vi "Main.vi"(11 "Module Admin":refnum<class "Delacor_lib_QMH_Cloneable Module Admin.lvclass">) -> ()   [LabVIEW 2021, in "TCP-IP Engine.lvlib"]
doc: "This template is based off of the Queued Message Handler design pattern and the Queued Message Handler project template that ships with LabVIEW.\n\nThe main difference is that the queue is private to this module and communication between modules is performed via Broadcast and Request events.\n\nRequest events are wrapped in public API methods and are handled in the Event Handling Loop (EHL) of this VI. Any module can register for Broadcast events sent by this module. The EHL generates messages based on user interface actions.\n\nThe Message Handling Loop (MHL) processes messages generated by the EHL, or by other messages. The messages are string values, so new messages can be added easily to the Message Cases case structure in the MHL. Each message cluster can also provide an optional value for Message Data, which is a variant that can be converted to whatever message-specific data is required.\n_____\nBased on DQMH Project Template 7.0.1.1316."
uses:
  TCP-IP Engine.lvlib
  <vilib>/Delacor/Delacor QMH/Libraries/Cloneable Module Admin_class/Delacor_lib_QMH_Cloneable Module Admin.lvclass
  C:/Program Files (x86)/National Instruments/LabVIEW 2024/vi.lib/Delacor/Delacor QMH/Libraries/Module Admin_class/Delacor_lib_QMH_Module Admin.lvclass
  Module Data--cluster.ctl
  TCP-Open Connection Argument--cluster.ctl
  <vilib>/Delacor/Delacor QMH/Libraries/Message Queue_class/Delacor_lib_QMH_Message Queue.lvclass/Delacor_lib_QMH_Message Queue.ctl
  <vilib>/Delacor/Delacor QMH/Libraries/Cloneable Module Admin_class/Delacor_lib_QMH_Cloneable Module Admin.lvclass/Delacor_lib_QMH_Cloneable Module Admin.ctl
  Stop Argument--cluster.ctl
  <vilib>/Delacor/Delacor QMH/Libraries/Module Admin_class/Delacor_lib_QMH_Module Admin.lvclass/Delacor_lib_QMH_Module Admin.ctl
  Read TCP Data Argument--cluster.ctl
  TCP-Write Argument--cluster.ctl
  TCP-Close Connection Argument--cluster.ctl
  <vilib>/Utility/miscctls.llb/LVPointTypeDef.ctl
  <vilib>/Delacor/Delacor QMH/Libraries/Message Queue_class/Delacor_lib_QMH_Enqueue Message (Single).vi
  <vilib>/Delacor/Delacor QMH/Libraries/Cloneable Module Admin_class/Delacor_lib_QMH_Get Module ID.vi
  <vilib>/Delacor/Delacor QMH/Libraries/Module Admin_class/Delacor_lib_QMH_Get External Launch.vi
  <vilib>/Delacor/Delacor QMH/Libraries/Message Queue_class/Delacor_lib_QMH_Message Queue.lvclass
panel:
  out "x >= y?":bool
  out "error out":errorcluster
  out "Status":string
  in  "Simulate EHL Error":bool
  in  "Simulate MHL Error":bool
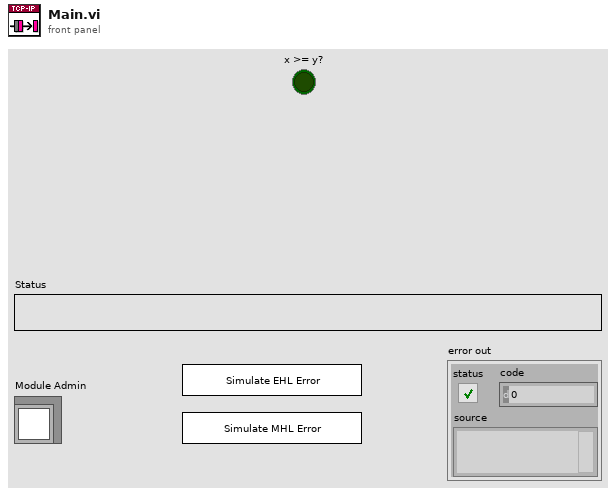
[diagram p1: front panel]
types:
  T1 = typedef "TCP-IP Engine.lvlib/Request Events--cluster.ctl" = cluster{"Stop Module":refnum<user-event>, "Show Panel":refnum<user-event>, "Hide Panel":refnum<user-event>, "Show Diagram":refnum<user-event>, "Get Module Execution Status":refnum<user-event>, "TCP-Open Connection":refnum<user-event>, "Read TCP Data":refnum<user-event>, "TCP-Write":refnum<user-event>, "TCP-Close Connection":refnum<user-event>}
  T2 = typedef "TCP-IP Engine.lvlib/Module Data--cluster.ctl" = cluster{"Status":string, "TCP-ID":refnum<k5>, "TCP-Open Connection Argument":T3, "OC Err Time":timestamp}
  T3 = typedef "TCP-IP Engine.lvlib/TCP-Open Connection Argument--cluster.ctl" = cluster{"Module ID":i32, "local port (0)":u16, "timeout ms (60000)":i32, "remote port ":u16, "address":string}
  T4 = enum32{"invalid lock state", "Not Locked", "Locked (No Password)", "Password-protected"}
  T5 = typedef "TCP-IP Engine.lvlib/Stop Argument--cluster.ctl" = cluster{"Module ID":i32, "Origin":string, "Exit via Stop Module Req?":bool, "Wait for Module to stop?":bool}
  T6 = typedef "TCP-IP Engine.lvlib/Read TCP Data Argument--cluster.ctl" = cluster{"Module ID":i32, "mode (standard)":enum16{"Standard", "Buffered", "CRLF", "Immediate"}, "timeout ms (25000)":i32, "bytes to read":i32}
  T7 = typedef "TCP-IP Engine.lvlib/TCP-Write Argument--cluster.ctl" = cluster{"Module ID":i32, "timeout ms (25000)":i32, "data in":string}
  T8 = typedef "TCP-IP Engine.lvlib/TCP-Close Connection Argument--cluster.ctl" = cluster{"Module ID":i32, "abort (F)":bool}
  T9 = typedef "LVPointTypeDef.ctl" = cluster{"Horizontal":i16, "Vertical":i16}
  T10 = enum32{"Invalid", "Standard", "Closed", "Hidden", "Minimized", "Maximized"}
  T11 = enum16{"big-endian, network order", "native, host order", "little-endian"}
  T12 = enum16{"Standard", "Buffered", "CRLF", "Immediate"}
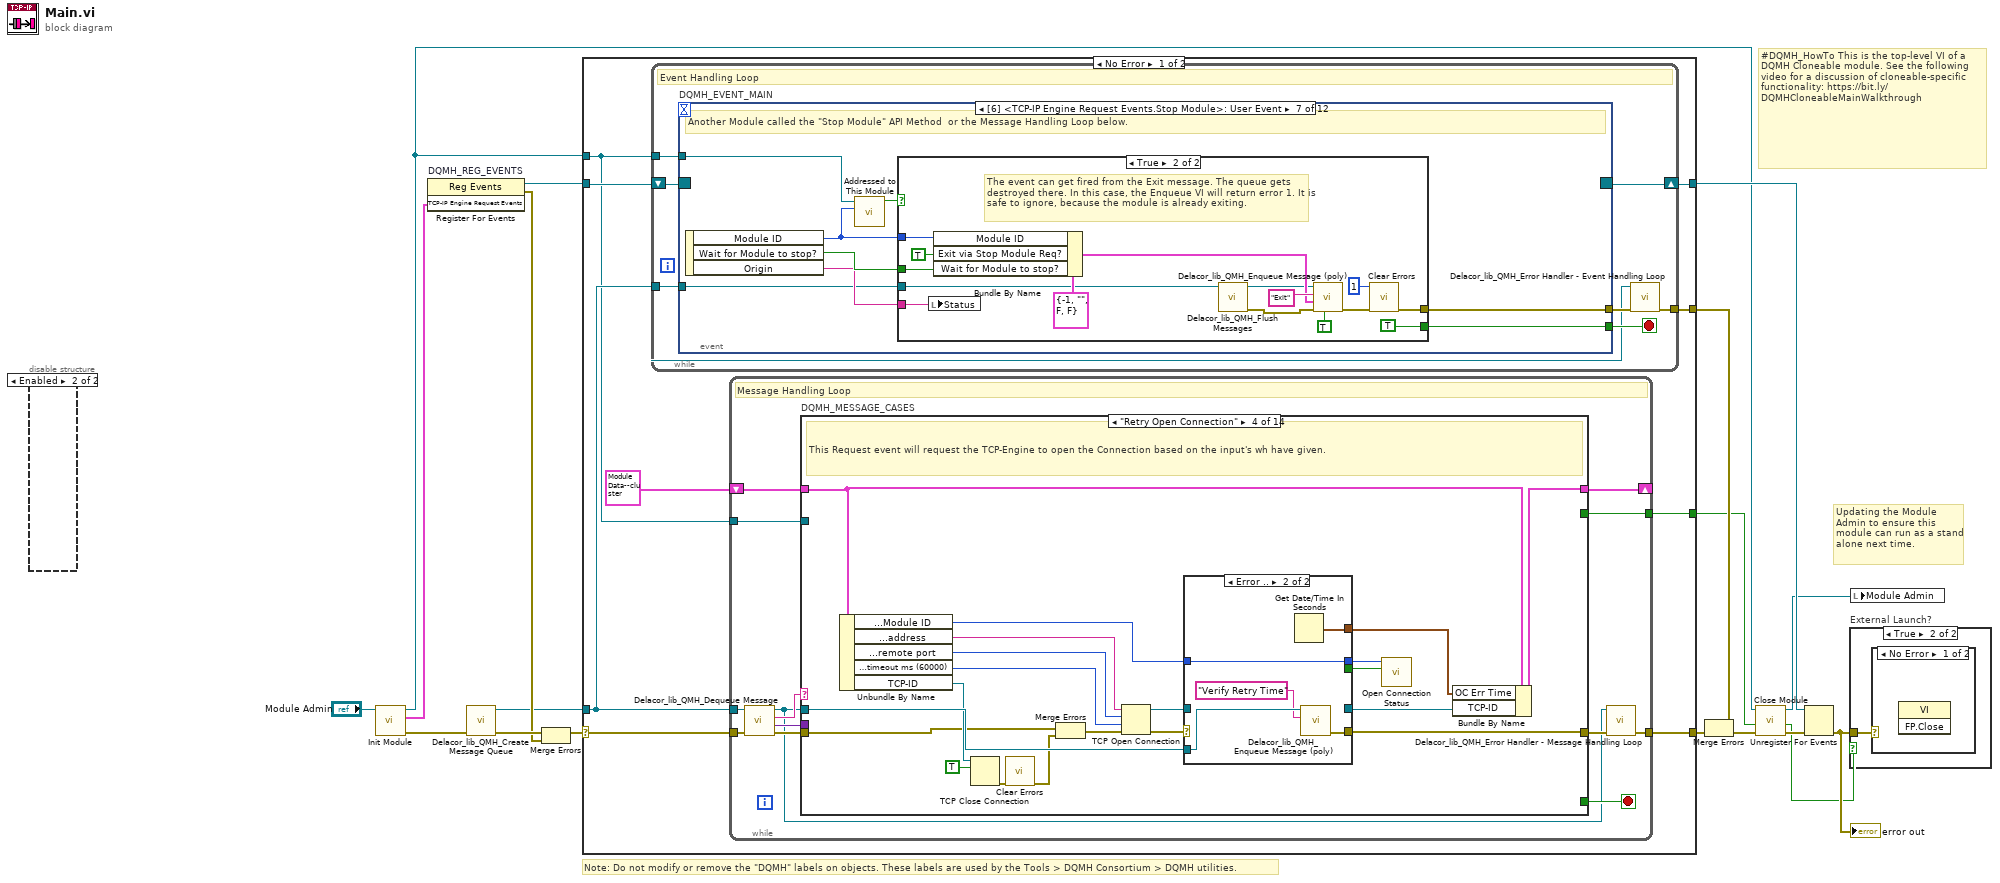
[diagram p0: block diagram]
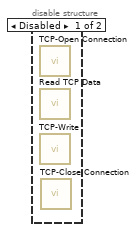
[diagram p2: hidden frame]
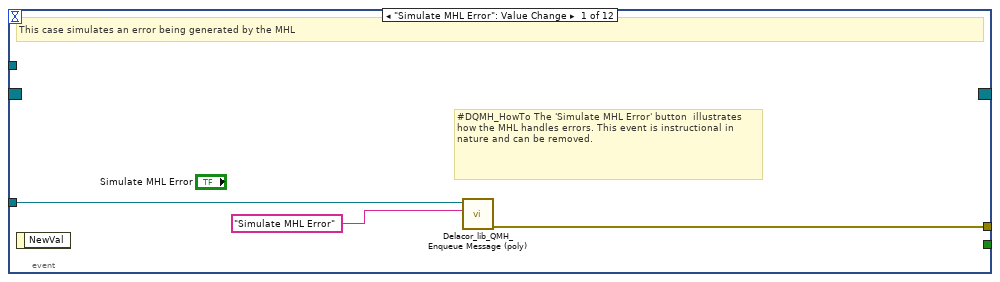
[diagram p3: hidden frame]
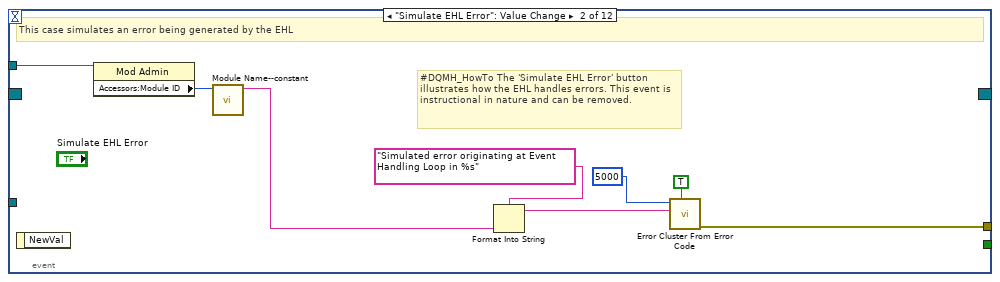
[diagram p4: hidden frame]
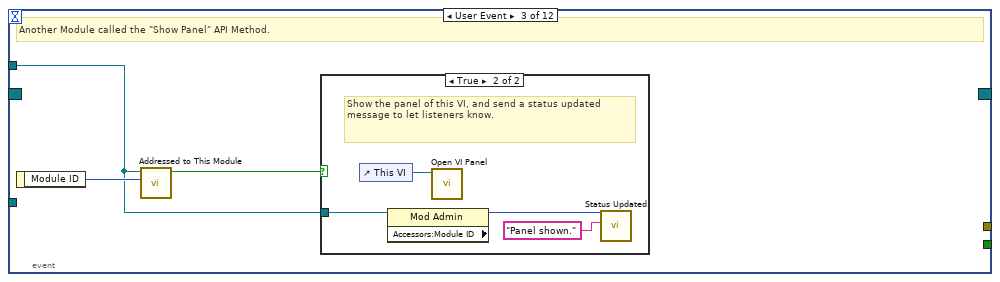
[diagram p5: hidden frame]
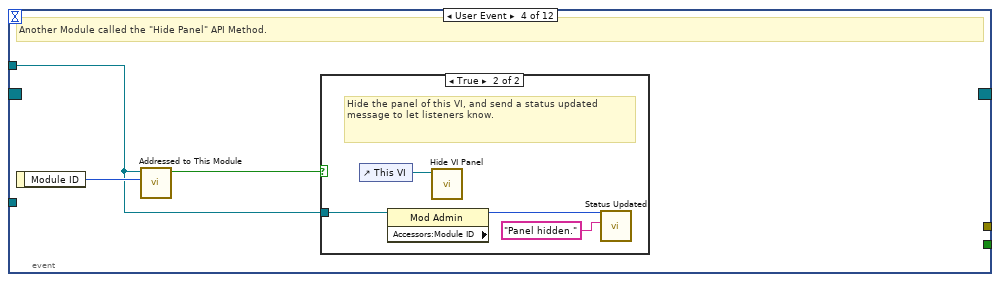
[diagram p7: hidden frame]
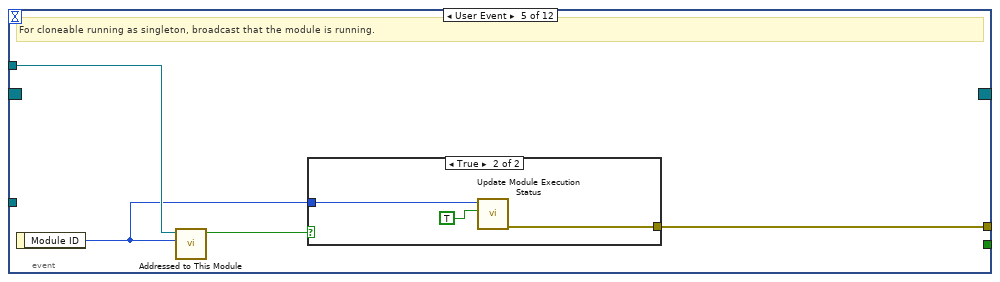
[diagram p9: hidden frame]
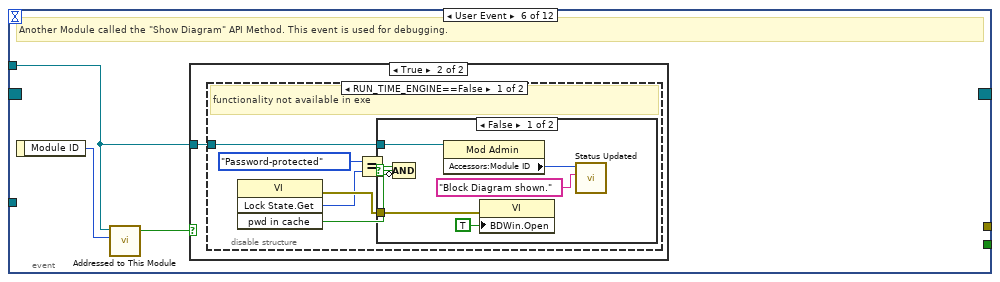
[diagram p11: hidden frame]
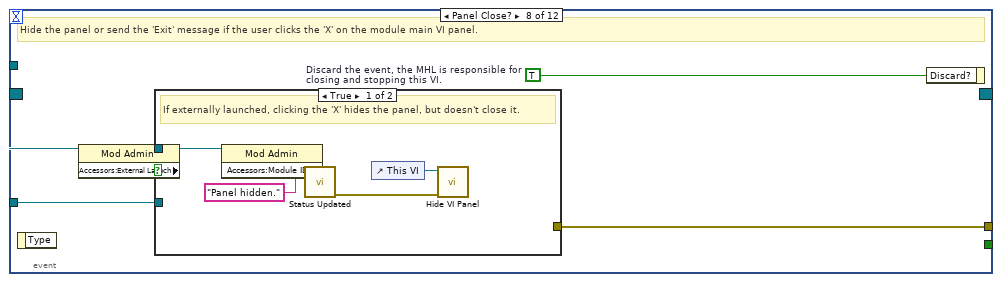
[diagram p16: hidden frame]
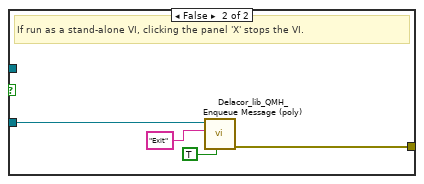
[diagram p17: hidden frame]
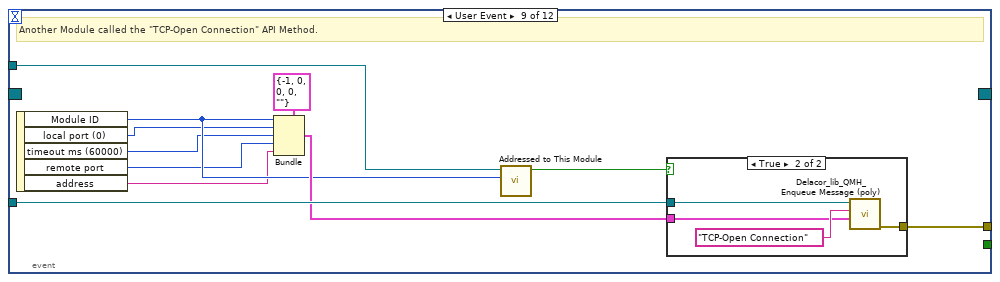
[diagram p18: hidden frame]
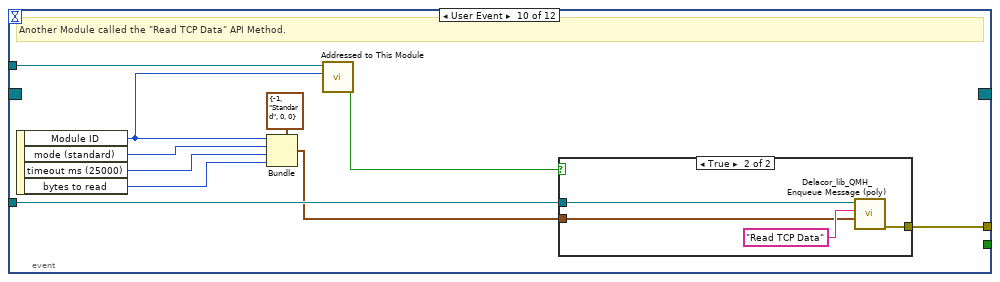
[diagram p20: hidden frame]
diagram:
  # "#DQMH_HowTo This is the top-level VI of a DQMH Cloneable module. See the following video for a discussion of cloneable-specific functionality: https://bit.ly/DQMHCloneableMainWalkthrough"
  # "Note: Do not modify or remove the \"DQMH\" labels on objects. These labels are used by the Tools > DQMH Consortium > DQMH utilities."
  # "Updating the Module Admin to ensure this module can run as a stand alone next time."
  n1 = disable-structure shown="Enabled" {
    frame Disabled {
      n2 = call "TCP-Open Connection.vi"() -> ()  [unwired: 11 in, 1 out]
      n3 = call "Read TCP Data.vi"() -> ()  [unwired: 11 in, 1 out]
      n4 = call "TCP-Write.vi"() -> ()  [unwired: 11 in, 1 out]
      n5 = call "TCP-Close Connection.vi"() -> ()  [unwired: 11 in, 1 out]
    }
    frame Enabled {
    }
  }
  n6 = call "Init Module.vi"("Cloneable Module Admin in"="Module Admin") -> ("error out"=w15:errorcluster, "TCP-IP Engine Request Events"=w7:T1, "Cloneable Module Admin out"=w4:refnum<class "Delacor_lib_QMH_Cloneable Module Admin.lvclass">)  [unwired: 8 in]
  n7 = register-events "DQMH_REG_EVENTS"(w7) -> (reference out=w8:refnum<event-registration>, error out=w10:errorcluster)  [unwired: 2 in]
  n8 = call <vilib>:"Delacor_lib_QMH_Create Message Queue.vi"("error in"=w15) -> ("error out"=w12:errorcluster, "Message Queue"=w6:refnum<class "Delacor_lib_QMH_Message Queue.lvclass">)  [unwired: 9 in]
  n9 = Merge Errors(w12, w10) -> (w11:errorcluster)
  n10 = case shown="No Error" w11 {
    selector: w11 -> [w25 w458]
    tunnel: [w27 w457] -> w16
    tunnel: [w24 w456] -> w9
    tunnel: w8 -> [w22 w456]
    tunnel: w6 -> [w21 w449]
    tunnel: [w26 _] -> w17
    tunnel: w4 -> [w20 w452]
    tunnel: [w19 _] -> w2
    frame No Error {
      n11 = while {
        tunnel: w21 -> [w28]
        shift-right: [w31] -> w24
        shift-left: w22 -> [w32]
        tunnel: [w33] -> w26
        tunnel: w20 -> [w29]
        stop <- w30 stop-if-true
        # "Event Handling Loop"
        n12 = event "DQMH_EVENT_MAIN" shown="[6] <TCP-IP Engine Request Events.Stop Module>: User Event" {
          selector: w32 -> [_ _ _ _ _ _ _ _ _ _ _ _]
          dyn-events: [_ _ _ _ _ _ _ _ _ _ _ _] -> w31
          timeout: _ -> [_ _ _ _ _ _ _ _ _ _ _ _]
          tunnel: [_ _ _ _ _ _ w87 _ _ _ _ _] -> w30
          tunnel: w28 -> [w36 _ _ _ _ _ w83 w108 w131 w145 w158 w171]
          tunnel: [w37 w45 _ _ w63 _ w90 w111 w121 w136 w150 w164] -> w34
          tunnel: w29 -> [_ w44 w46 w53 w61 w67 w89 w109 w129 w143 w156 w169]
          event "Simulate MHL Error": Value Change {
            # "#DQMH_HowTo The 'Simulate MHL Error' button  illustrates how the MHL handles errors. This event is instructional in nature and can be removed."
            # "This case simulates an error being generated by the MHL"
            n13 = event-data() -> ()  [unwired: 1 in, 1 out]
            n14 = call-poly <vilib>:"Delacor_lib_QMH_Enqueue Message (poly).vi"("Message"="Simulate MHL Error", "Message Queue in"=w36) -> ("error out"=w37:errorcluster)  [unwired: 8 in, 1 out]
          }
          event "Simulate EHL Error": Value Change {
            # "#DQMH_HowTo The 'Simulate EHL Error' button  illustrates how the EHL handles errors. This event is instructional in nature and can be removed."
            # "This case simulates an error being generated by the EHL"
            n15 = event-data() -> ()  [unwired: 1 in, 1 out]
            n16 = property on="Property Node" class="Mod Admin"(reference=w44) -> ("Accessors:Module ID"=w43:i32)  [unwired: 1 in, 2 out]
            n17 = call "Module Name--constant.vi"("Module ID"=w43) -> ("Module Name"=w38:string)  [unwired: 10 in]
            n18 = Format Into String(format string="Simulated error originating at Event Handling Loop in %s", w38) -> (resulting string=w41:string)  [unwired: 2 in, 1 out]
            n19 = call <vilib>:"Error Cluster From Error Code.vi"("show call chain? (False)"=TRUE, "error message (\"\")"=w41, "error code (0)"=5000) -> ("error out"=w45:errorcluster)  [unwired: 6 in]
          }
          event User Event {
            # "Another Module called the \"Show Panel\" API Method."
            n20 = event-data() -> ("Module ID"=w47:i32)  [unwired: 1 in]
            n21 = call "Addressed to This Module.vi"("Module ID from Argument"=w47, "Module Admin"=w46) -> ("Addressed to this instance?"=w48:bool)  [unwired: 8 in, 1 out]
            n22 = case shown="True" w48 {
              tunnel: w46 -> [_ w50]
              frame False {
              }
              frame True {
                # "Show the panel of this VI, and send a status updated message to let listeners know."
                n23 = control-ref of="This VI"() -> (w52:refnum<vi>)
                n24 = property on="Property Node" class="Mod Admin"(reference=w50) -> ("Accessors:Module ID"=w49:i32)  [unwired: 1 in, 2 out]
                n25 = call "Open VI Panel.vi"("VI"=w52) -> ()  [unwired: 10 in, 1 out]
                n26 = call "Status Updated.vi"("Status"="Panel shown." ("format string"), "Module ID"=w49) -> ()  [unwired: 9 in, 1 out]
              }
            }
          }
          event User Event {
            # "Another Module called the \"Hide Panel\" API Method."
            n27 = event-data() -> ("Module ID"=w54:i32)  [unwired: 1 in]
            n28 = call "Addressed to This Module.vi"("Module ID from Argument"=w54, "Module Admin"=w53) -> ("Addressed to this instance?"=w55:bool)  [unwired: 8 in, 1 out]
            n29 = case shown="True" w55 {
              tunnel: w53 -> [_ w57]
              frame False {
              }
              frame True {
                # "Hide the panel of this VI, and send a status updated message to let listeners know."
                n30 = control-ref of="This VI"() -> (w59:refnum<vi>)
                n31 = property on="Property Node" class="Mod Admin"(reference=w57) -> ("Accessors:Module ID"=w56:i32)  [unwired: 1 in, 2 out]
                n32 = call "Hide VI Panel.vi"("VI"=w59) -> ()  [unwired: 10 in, 1 out]
                n33 = call "Status Updated.vi"("Status"="Panel hidden." ("format string"), "Module ID"=w56) -> ()  [unwired: 9 in, 1 out]
              }
            }
          }
          event User Event {
            # "For cloneable running as singleton, broadcast that the module is running."
            n34 = event-data() -> ("Module ID"=w60:i32)  [unwired: 1 in]
            n35 = call "Addressed to This Module.vi"("Module ID from Argument"=w60, "Module Admin"=w61) -> ("Addressed to this instance?"=w62:bool)  [unwired: 8 in, 1 out]
            n36 = case shown="True" w62 {
              tunnel: [_ w66] -> w63
              tunnel: w60 -> [_ w65]
              frame False {
              }
              frame True {
                n37 = call "Update Module Execution Status.vi"("Running?"=TRUE, "Module ID"=w65) -> ("error out"=w66:errorcluster)  [unwired: 9 in]
              }
            }
          }
          event User Event {
            # "Another Module called the \"Show Diagram\" API Method. This event is used for debugging."
            n38 = event-data() -> ("Module ID"=w68:i32)  [unwired: 1 in]
            n39 = call "Addressed to This Module.vi"("Module ID from Argument"=w68, "Module Admin"=w67) -> ("Addressed to this instance?"=w69:bool)  [unwired: 8 in, 1 out]
            n40 = case shown="True" w69 {
              tunnel: w67 -> [_ w70]
              frame False {
              }
              frame True {
                n41 = disable-structure shown="RUN_TIME_ENGINE==False" {
                  disable-tunnel: w70 -> [w71 _]
                  frame condition #0 (active) {
                    # "functionality not available in exe"
                    n42 = invoke on="Invoke Node" class="VI" method="Lock State.Get"() -> (error out=w77:errorcluster, "Get Lock State"=w76:T4, "pwd in cache"=w73:bool)  [unwired: 4 in, 1 out]
                    n43 = Equal?(x=T4."Password-protected", y=w76) -> (x = y?=w74:bool)
                    n44 = Compound Arithmetic op=AND(w74, invert w73) -> (w72:bool)
                    n45 = case shown="False" w72 {
                      tunnel: w77 -> [w82 _]
                      tunnel: w71 -> [w79 _]
                      frame False {
                        n46 = property on="Property Node" class="Mod Admin"(reference=w79) -> ("Accessors:Module ID"=w78:i32)  [unwired: 1 in, 2 out]
                        n47 = property on="Property Node" class="VI"(error in=w82, "BDWin.Open"=TRUE ("Block Diagram Window:Open")) -> ()  [unwired: 1 in, 2 out]
                        n48 = call "Status Updated.vi"("Status"="Block Diagram shown." ("format string"), "Module ID"=w78) -> ()  [unwired: 9 in, 1 out]
                      }
                      frame True {
                        # "Password-protected VI, and the password is not in the cache. Do not show the diagram."
                      }
                    }
                  }
                  frame condition #1 {
                  }
                }
              }
            }
          }
          event User Event {
            # "Another Module called the \"Stop Module\" API Method  or the Message Handling Loop below."
            n49 = event-data() -> ("Module ID"=w85:i32, "Wait for Module to stop?"=w86:bool, "Origin"=w84:string)  [unwired: 1 in]
            n50 = call "Addressed to This Module.vi"("Module ID from Argument"=w85, "Module Admin"=w89) -> ("Addressed to this instance?"=w88:bool)  [unwired: 8 in, 1 out]
            n51 = case shown="True" w88 {
              tunnel: [_ w104] -> w90
              tunnel: w83 -> [_ w93]
              tunnel: [_ TRUE] -> w87
              tunnel: w86 -> [_ w96]
              tunnel: w85 -> [_ w98]
              tunnel: w84 -> [_ w94]
              frame False {
              }
              frame True {
                # "The event can get fired from the Exit message. The queue gets destroyed there. In this case, the Enqueue VI will return error 1. It is safe to ignore, because the module is already exiting."
                n52 = local write "Status"(w94) -> ()
                n53 = Bundle By Name(cluster=T5 {"Module ID"=-1, "Origin"="", "Exit via Stop Module Req?"=FALSE, "Wait for Module to stop?"=FALSE} ("Stop Argument"), "Module ID"=w98, "Exit via Stop Module Req?"=TRUE, "Wait for Module to stop?"=w96) -> (w95:T5)
                n54 = call-dynamic "Delacor_lib_QMH_Flush Messages.vi"("Message Queue in"=w93) -> ("error out"=w91:errorcluster, "Message Queue out"=w92:refnum<class "Delacor_lib_QMH_Message Queue.lvclass">)  [unwired: 7 in, 2 out]
                n55 = call-poly <vilib>:"Delacor_lib_QMH_Enqueue Message (poly).vi"("Priority Message? (F)"=TRUE, "error in"=w91, "Message Data"=w95, "Message"="Exit", "Message Queue in"=w92) -> ("error out"=w105:errorcluster)  [unwired: 5 in, 1 out]
                n56 = call <vilib>:"Clear Errors.vi"("error in (no error)"=w105, "specific error code to clear (0: all)"=1) -> ("error out"=w104:errorcluster)  [unwired: 4 in, 1 out]
              }
            }
          }
          event Panel Close? {
            w110 = TRUE  # Discard the event, the MHL is responsible for closing and stopping this VI.
            # "Hide the panel or send the 'Exit' message if the user clicks the 'X' on the module main VI panel."
            n57 = event-data() -> ()  [unwired: 1 in, 1 out]
            n58 = property on="Property Node" class="Mod Admin"(reference=w109) -> (reference out=w106:refnum<class "Delacor_lib_QMH_Cloneable Module Admin.lvclass">, "Accessors:External Launch"=w107:bool)  [unwired: 1 in, 1 out]
            n59 = case shown="True" w107 {
              tunnel: w108 -> [_ w119]
              tunnel: [_ w120] -> w111
              tunnel: w106 -> [w114 _]
              frame True {
                # "If externally launched, clicking the 'X' hides the panel, but doesn't close it."
                n60 = property on="Property Node" class="Mod Admin"(reference=w114) -> ("Accessors:Module ID"=w113:i32)  [unwired: 1 in, 2 out]
                n61 = call "Status Updated.vi"("Status"="Panel hidden." ("format string"), "Module ID"=w113) -> ("error out"=w112:errorcluster)  [unwired: 9 in]
                n62 = control-ref of="This VI"() -> (w116:refnum<vi>)
                n63 = call "Hide VI Panel.vi"("error in"=w112, "VI"=w116) -> ()  [unwired: 9 in, 1 out]
              }
              frame False {
                # "If run as a stand-alone VI, clicking the panel 'X' stops the VI."
                n64 = call-poly <vilib>:"Delacor_lib_QMH_Enqueue Message (poly).vi"("Priority Message? (F)"=TRUE, "Message"="Exit", "Message Queue in"=w119) -> ("error out"=w120:errorcluster)  [unwired: 7 in, 1 out]
              }
            }
            n65 = event-data ("Event Filter Node")("Discard?"=w110) -> ()  [unwired: 1 in, 1 out]
          }
          event User Event {
            # "Another Module called the \"TCP-Open Connection\" API Method."
            n66 = event-data() -> ("Module ID"=w126:i32, "local port (0)"=w125:u16, "timeout ms (60000)"=w124:i32, "remote port"=w123:u16, "address"=w122:string)  [unwired: 1 in]
            n67 = Bundle(cluster=T3 {"Module ID"=-1, "local port (0)"=0, "timeout ms (60000)"=0, "remote port "=0, "address"=""} ("TCP-Open Connection Argument"), "Module ID"=w126, "local port (0)"=w125, "timeout ms (60000)"=w124, "remote port"=w123, "address"=w122) -> (w127:T3)
            n68 = call "Addressed to This Module.vi"("Module ID from Argument"=w126, "Module Admin"=w129) -> ("Addressed to this instance?"=w130:bool)  [unwired: 8 in, 1 out]
            n69 = case shown="True" w130 {
              tunnel: w131 -> [_ w135]
              tunnel: w127 -> [_ w133]
              tunnel: [_ w132] -> w121
              frame False {
              }
              frame True {
                n70 = call-poly <vilib>:"Delacor_lib_QMH_Enqueue Message (poly).vi"("Message Data"=w133, "Message"="TCP-Open Connection", "Message Queue in"=w135) -> ("error out"=w132:errorcluster)  [unwired: 7 in, 1 out]
              }
            }
          }
          event User Event {
            # "Another Module called the \"Read TCP Data\" API Method."
            n71 = event-data() -> ("Module ID"=w140:i32, "mode (standard)"=w139:T12, "timeout ms (25000)"=w138:i32, "bytes to read"=w137:i32)  [unwired: 1 in]
            n72 = Bundle(cluster=T6 {"Module ID"=-1, "mode (standard)"=enum."Standard", "timeout ms (25000)"=0, "bytes to read"=0} ("Read TCP Data Argument"), "Module ID"=w140, "mode (standard)"=w139, "timeout ms (25000)"=w138, "bytes to read"=w137) -> (w141:T6)
            n73 = call "Addressed to This Module.vi"("Module ID from Argument"=w140, "Module Admin"=w143) -> ("Addressed to this instance?"=w144:bool)  [unwired: 8 in, 1 out]
            n74 = case shown="True" w144 {
              tunnel: w145 -> [_ w149]
              tunnel: w141 -> [_ w147]
              tunnel: [_ w146] -> w136
              frame False {
              }
              frame True {
                n75 = call-poly <vilib>:"Delacor_lib_QMH_Enqueue Message (poly).vi"("Message Data"=w147, "Message"="Read TCP Data", "Message Queue in"=w149) -> ("error out"=w146:errorcluster)  [unwired: 7 in, 1 out]
              }
            }
          }
          event User Event {
            # "Another Module called the \"TCP-Write\" API Method."
            n76 = event-data() -> ("Module ID"=w153:i32, "timeout ms (25000)"=w152:i32, "data in"=w151:string)  [unwired: 1 in]
            n77 = Bundle(cluster=T7 {"Module ID"=-1, "timeout ms (25000)"=0, "data in"=""} ("TCP-Write Argument"), "Module ID"=w153, "timeout ms (25000)"=w152, "data in"=w151) -> (w154:T7)
            n78 = call "Addressed to This Module.vi"("Module ID from Argument"=w153, "Module Admin"=w156) -> ("Addressed to this instance?"=w157:bool)  [unwired: 8 in, 1 out]
            n79 = case shown="True" w157 {
              tunnel: w158 -> [_ w163]
              tunnel: w154 -> [_ w161]
              tunnel: [_ w160] -> w150
              frame False {
              }
              frame True {
                n80 = call-poly <vilib>:"Delacor_lib_QMH_Enqueue Message (poly).vi"("Priority Message? (F)"=TRUE, "Message Data"=w161, "Message"="TCP-Write", "Message Queue in"=w163) -> ("error out"=w160:errorcluster)  [unwired: 6 in, 1 out]
              }
            }
          }
          event User Event {
            # "Another Module called the \"TCP-Close Connection\" API Method."
            n81 = event-data() -> ("Module ID"=w166:i32, "abort (F)"=w165:bool)  [unwired: 1 in]
            n82 = Bundle(cluster=T8 {"Module ID"=-1, "abort (F)"=FALSE} ("TCP-Close Connection Argument"), "Module ID"=w166, "abort (F)"=w165) -> (w167:T8)
            n83 = call "Addressed to This Module.vi"("Module ID from Argument"=w166, "Module Admin"=w169) -> ("Addressed to this instance?"=w170:bool)  [unwired: 8 in, 1 out]
            n84 = case shown="True" w170 {
              tunnel: w171 -> [_ w175]
              tunnel: w167 -> [_ w173]
              tunnel: [_ w172] -> w164
              frame False {
              }
              frame True {
                n85 = call-poly <vilib>:"Delacor_lib_QMH_Enqueue Message (poly).vi"("Message Data"=w173, "Message"="TCP-Close Connection", "Message Queue in"=w175) -> ("error out"=w172:errorcluster)  [unwired: 7 in, 1 out]
              }
            }
          }
        }
        n86 = call-dynamic "Delacor_lib_QMH_Error Handler - Event Handling Loop.vi"("error in"=w34, "Message Queue in"=w28) -> ("dup error in"=w33:errorcluster)  [unwired: 8 in, 1 out]
      }
      n87 = while {
        tunnel: w21 -> [w176]
        shift-right: [w183] -> _
        shift-left: T2 {"Status"="", "TCP-ID"=refnum, "TCP-Open Connection Argument"={"Module ID"=-1, "local port (0)"=0, "timeout ms (60000)"=0, "remote port "=0, "address"=""}, "OC Err Time"=timestamp(0 s since 1904-01-01)} ("Data Cluster") -> [w184]
        tunnel: w25 -> [w187]
        tunnel: [w185] -> w27
        tunnel: w20 -> [w178]
        tunnel: [w177] -> w19
        stop <- w182 stop-if-true
        # "Message Handling Loop"
        n88 = call-dynamic "Delacor_lib_QMH_Dequeue Message.vi"("error in"=w187, "Message Queue in"=w176) -> ("error out"=w186:errorcluster, "Message Data"=w180:variant, "Message"=w181:string, "Message Queue out"=w179:refnum<class "Delacor_lib_QMH_Message Queue.lvclass">)  [unwired: 6 in]
        n89 = case "DQMH_MESSAGE_CASES" shown="\"Retry Open Connection\"" w181 {
          selector: w181 -> [_ _ _ _ _ _ _ _ _ _ _ _ _ w438]
          tunnel: w179 -> [_ _ w213 w247 w276 _ _ _ w369 _ w390 _ w430 _]
          tunnel: w186 -> [w207 w211 w230 w242 w288 w349 w363 w366 w370 w387 w399 w416 w436 w447]
          tunnel: [w205 w211 w220 w254 w283 w343 w358 w365 w378 w387 w395 w415 w431 w448] -> w188
          tunnel: w184 -> [w198 w210 w223 w248 w279 w345 w356 w364 w377 w386 w394 w413 w420 w445]
          tunnel: [w197 w210 w222 w256 w278 w344 w356 w364 w377 w386 w394 w413 w420 w445] -> w183
          tunnel: [_ _ _ _ _ _ _ _ _ _ _ _ w429 _] -> w182
          tunnel: w180 -> [_ _ w229 _ w287 w348 w362 _ _ _ w393 _ w427 _]
          tunnel: w178 -> [w192 _ _ _ _ _ _ _ _ _ w392 w411 w422 w444]
          tunnel: [_ _ _ _ _ _ _ _ _ _ _ _ w425 _] -> w177
          frame "Initialize" {
            w189 = "Initial Message" ("Initial Message")
            # "#CodeNeeded - Initialize the appearance of the front panel."
            # "#CodeNeeded - Initialize your state data here."
            # "Initialize - Any operation that needs to be done before the module can receive messages. Synchronize Caller Events.vi will inform Start Module.vi that the module has launched and is ready to receive messages. Module Did Init.vi will broadcast that the module initialized."
            n90 = call "Synchronize Caller Events.vi"("error in"=w207, "Module Admin"=w192) -> ("error out"=w206:errorcluster, "Module Admin out"=w191:refnum<class "Delacor_lib_QMH_Cloneable Module Admin.lvclass">)  [unwired: 8 in]
            n91 = property on="Property Node" class="Mod Admin"(reference=w191) -> ("Accessors:Module ID"=w194:i32, "Accessors:External Launch"=w193:bool)  [unwired: 1 in, 2 out]
            n92 = call "Module Name--constant.vi"("Module ID"=w194) -> ("Module Name"=w202:string)  [unwired: 10 in]
            n93 = property on="Property Node" class="VI"("Front Panel.Title"=w202) -> (reference out=w204:refnum<vi>, error out=w209:errorcluster)  [unwired: 2 in]
            n94 = Select(t=T10."Hidden" ("State"), s=w193, f=T10."Standard" ("State")) -> (s? t:f=w199:T10)
            n95 = invoke on="Invoke Node" class="VI" method="FP.Open"(reference=w204, error in=w209, "State"=w199) -> (reference out=w203:refnum<vi>, error out=w208:errorcluster)  [unwired: 2 in, 3 out]
            n96 = call "Module Name--constant.vi"("Module ID"=w194) -> ("Module Name"=w195:string)  [unwired: 10 in]
            n97 = Bundle By Name(cluster=w198, "Status"=w189) -> (w197:T2)
            n98 = invoke on="Invoke Node" class="VI" method="FP.Center"(reference=w203, error in=w208) -> ()  [unwired: 1 in, 3 out]
            n99 = property on="Pane" class="Pane"("Origin"=T9 {"Horizontal"=0, "Vertical"=0}) -> ()  [unwired: 2 in, 2 out]
            n100 = call "Module Did Init.vi"("error in"=w206, "Initialized?"=TRUE, "Origin"=w195, "Module ID"=w194) -> ("error out"=w205:errorcluster)  [unwired: 7 in]
            "Status" <- w189
          }
          frame "---Module Specific---" {
            # "Separator -- The following cases handle messages specific to this Module."
          }
          frame "TCP-Open Connection" {
            # "This Request event will request the TCP-Engine to open the Connection based on the input's wh have given."
            n101 = Variant To Data(error in=w230, type=T3 {"Module ID"=-1, "local port (0)"=0, "timeout ms (60000)"=0, "remote port "=0, "address"=""} ("TCP-Open Connection Argument"), Variant=w229) -> (data=w214:T3, error out=w227:errorcluster)
            n102 = Unbundle By Name(w214) -> ("Module ID"=w217:i32, "address"=w224:string, "remote port"=w225:u16, "timeout ms (60000)"=w226:i32)
            n103 = TCP Open Connection(address=w224, remote port or service name=w225, timeout ms (60000)=w226, error in (no error)=w227) -> (connection ID=w219:refnum<k5>, error out=w221:errorcluster)  [unwired: 1 in]
            n104 = case shown="Error .." w221 {
              selector: w221 -> [w234 _]
              tunnel: [w234 w237] -> w220
              tunnel: w219 -> [w233 _]
              tunnel: [w233 _] -> w218
              tunnel: w217 -> [w232 w239]
              tunnel: [w232 w239] -> w216
              tunnel: [TRUE _] -> w215
              tunnel: w213 -> [_ w236]
              tunnel: [_ w235] -> w212
              frame No Error {
              }
              frame Error {
                n105 = Get Date/Time In Seconds() -> (seconds since 1Jan1904=w235:timestamp)
                n106 = call-poly <vilib>:"Delacor_lib_QMH_Enqueue Message (poly).vi"("Message"="Verify Retry Time", "Message Queue in"=w236) -> ("error out"=w237:errorcluster)  [unwired: 8 in, 1 out]
              }
            }
            n107 = call "Open Connection Status.vi"("Connection Status?"=w215, "Module ID"=w216) -> ()  [unwired: 9 in, 1 out]
            n108 = Bundle By Name(cluster=w223, "OC Err Time"=w212, "TCP-Open Connection Argument"=w214, "TCP-ID"=w218) -> (w222:T2)
          }
          frame "Retry Open Connection" {
            # "This Request event will request the TCP-Engine to open the Connection based on the input's wh have given."
            n109 = Unbundle By Name(w248) -> ("TCP-Open Connection Argument.Module ID"=w251:i32, "TCP-Open Connection Argument.address"=w257:string, "TCP-Open Connection Argument.remote port"=w258:u16, "TCP-Open Connection Argument.timeout ms (60000)"=w259:i32, "TCP-ID"=w243:refnum<k5>)
            n110 = TCP Close Connection(connection ID=w243, abort (F)=TRUE) -> (error out=w244:errorcluster)  [unwired: 1 in, 1 out]
            n111 = call <vilib>:"Clear Errors.vi"("error in (no error)"=w244) -> ("error out"=w241:errorcluster)  [unwired: 5 in, 1 out]
            n112 = Merge Errors(w242, w241) -> (w240:errorcluster)
            n113 = TCP Open Connection(address=w257, remote port or service name=w258, timeout ms (60000)=w259, error in (no error)=w240) -> (connection ID=w253:refnum<k5>, error out=w255:errorcluster)  [unwired: 1 in]
            n114 = case shown="Error .." w255 {
              selector: w255 -> [w263 _]
              tunnel: [w263 w266] -> w254
              tunnel: w253 -> [w260 _]
              tunnel: [w260 _] -> w252
              tunnel: w251 -> [w262 w268]
              tunnel: [w262 w268] -> w250
              tunnel: [TRUE _] -> w249
              tunnel: w247 -> [_ w267]
              tunnel: [_ w265] -> w246
              frame No Error {
              }
              frame Error {
                n115 = Get Date/Time In Seconds() -> (seconds since 1Jan1904=w265:timestamp)
                n116 = call-poly <vilib>:"Delacor_lib_QMH_Enqueue Message (poly).vi"("Message"="Verify Retry Time", "Message Queue in"=w267) -> ("error out"=w266:errorcluster)  [unwired: 8 in, 1 out]
              }
            }
            n117 = call "Open Connection Status.vi"("Connection Status?"=w249, "Module ID"=w250) -> ()  [unwired: 9 in, 1 out]
            n118 = Bundle By Name(cluster=w248, "OC Err Time"=w246, "TCP-ID"=w252) -> (w256:T2)
          }
          frame "Read TCP Data" {
            # "This Request Event will request the TCP-IP Module to read the data from the respective connection."
            n119 = Variant To Data(error in=w288, type=T6 {"Module ID"=-1, "mode (standard)"=enum."Standard", "timeout ms (25000)"=0, "bytes to read"=0} ("Read TCP Data Argument"), Variant=w287) -> (data=w285:T6, error out=w284:errorcluster)
            n120 = Unbundle By Name(w285) -> ("Module ID"=w277:i32, "mode (standard)"=w282:T12, "bytes to read"=w281:i32, "timeout ms (25000)"=w280:i32)
            n121 = Unbundle By Name(w279) -> ("TCP-ID"=w275:refnum<k5>)
            n122 = TCP Read(connection ID=w275, bytes to read=w281, error in (no error)=w284, 7:w282, 9:w280) -> (connection ID out=w271:refnum<k5>, data out=w273:string, error out=w272:errorcluster)
            n123 = Empty String/Path?(string/path=w273) -> (empty?=w274:bool)
            n124 = case shown="True" w274 {
              tunnel: w273 -> [w297 _]
              tunnel: w272 -> [w296 w308]
              tunnel: [w293 w307] -> w283
              tunnel: w271 -> [w295 w306]
              tunnel: [w294 w305] -> w270
              tunnel: w277 -> [w291 w304]
              tunnel: w276 -> [_ w303]
              tunnel: [_ w302] -> w269
              frame False {
                n125 = Unflatten From String(type=0, binary string=w297, byte order (0:big-endian, network order)=T11."little-endian", error in (no error)=w296) -> (value=w300:i32, error out=w299:errorcluster)  [unwired: 1 in, 1 out]
                n126 = TCP Read(connection ID=w295, bytes to read=w300, error in (no error)=w299) -> (connection ID out=w294:refnum<k5>, data out=w290:string, error out=w293:errorcluster)  [unwired: 2 in]
                n127 = call "TCP-Read Data Out.vi"("TCP-IP Data Out"=w290, "Module ID"=w291) -> ("error out"=w289:errorcluster)  [unwired: 9 in]
                n128 = call "Open Connection Status.vi"("error in"=w289, "Connection Status?"=TRUE, "Module ID"=w291) -> ()  [unwired: 8 in, 1 out]
              }
              frame True {
                n129 = case shown="Default" w308 {
                  selector: w308 -> [w312 w315 _ _]
                  tunnel: [w312 w316 w326 _] -> w307
                  tunnel: w306 -> [w311 w313 w331 w334]
                  tunnel: [w311 _ _ w334] -> w305
                  tunnel: w304 -> [w309 w321 w327 w332]
                  tunnel: w303 -> [_ w314 w325 _]
                  tunnel: [_ w320 w323 _] -> w302
                  frame No Error {
                    n130 = call "Open Connection Status.vi"("Connection Status?"=TRUE, "Module ID"=w309) -> ()  [unwired: 9 in, 1 out]
                  }
                  frame Default {
                    n131 = TCP Close Connection(connection ID=w313, abort (F)=TRUE, error in (no error)=w315) -> (error out=w318:errorcluster)  [unwired: 1 out]
                    n132 = call "Open Connection Status.vi"("Connection Status?"=FALSE, "Module ID"=w321) -> ()  [unwired: 9 in, 1 out]
                    n133 = call <vilib>:"Clear Errors.vi"("error in (no error)"=w318) -> ()  [unwired: 5 in, 2 out]
                    n134 = call-poly <vilib>:"Delacor_lib_QMH_Enqueue Message (poly).vi"("Message"="Verify Retry Time", "Message Queue in"=w314) -> ("error out"=w316:errorcluster)  [unwired: 8 in, 1 out]
                    n135 = Get Date/Time In Seconds() -> (seconds since 1Jan1904=w320:timestamp)
                  }
                  frame Error {
                    n136 = TCP Close Connection(connection ID=w331, abort (F)=TRUE) -> (error out=w328:errorcluster)  [unwired: 1 in, 1 out]
                    n137 = call "Open Connection Status.vi"("Connection Status?"=FALSE, "Module ID"=w327) -> ()  [unwired: 9 in, 1 out]
                    n138 = call <vilib>:"Clear Errors.vi"("error in (no error)"=w328) -> ()  [unwired: 5 in, 2 out]
                    n139 = Get Date/Time In Seconds() -> (seconds since 1Jan1904=w323:timestamp)
                    n140 = call-poly <vilib>:"Delacor_lib_QMH_Enqueue Message (poly).vi"("Message"="Verify Retry Time", "Message Queue in"=w325) -> ("error out"=w326:errorcluster)  [unwired: 8 in, 1 out]
                  }
                  frame Error {
                    n141 = call "Open Connection Status.vi"("Connection Status?"=TRUE, "Module ID"=w332) -> ()  [unwired: 9 in, 1 out]
                  }
                }
              }
            }
            n142 = Bundle By Name(cluster=w279, "OC Err Time"=w269, "TCP-ID"=w270) -> (w278:T2)
          }
          frame "TCP-Write" {
            # "This Request event will request the TCP-IP Module to write the Data which is connected to the Data In terminal of the Input."
            n143 = Variant To Data(error in=w349, type=T7 {"Module ID"=-1, "timeout ms (25000)"=0, "data in"=""} ("TCP-Write Argument"), Variant=w348) -> (data=w346:T7, error out=w338:errorcluster)
            n144 = Unbundle By Name(w346) -> ("data in"=w337:string, "timeout ms (25000)"=w342:i32)  [unwired: 1 out]
            n145 = String Length(string=w337) -> (length=w341:i32)
            n146 = Flatten To String(anything=w341, byte order (0:big-endian, network order)=T11."little-endian", error in (no error)=w338) -> (data string=w339:string, error out=w335:errorcluster)  [unwired: 1 in, 1 out]
            n147 = Concatenate Strings(w339, w337) -> (w336:string)
            n148 = in-place {
              in-place-border: [w355] -> w343
              in-place-border: w342 -> [w354]
              in-place-border: w336 -> [w353]
              in-place-border: w335 -> [w350]
              n149 = in-place-cluster #1(w345) -> ("TCP-ID"=w352:refnum<k5>)
              n150 = TCP Write(connection ID=w352, data in=w353, error in (no error)=w350, 9:w354) -> (connection ID out=w351:refnum<k5>, error out=w355:errorcluster)  [unwired: 1 out]
              n151 = in-place-cluster #1("TCP-ID"=w351) -> (w344:T2)
            }
          }
          frame "TCP-Close Connection" {
            # "This Request Event will request the TCP-IP module to close the respective opened connection."
            n152 = Variant To Data(error in=w363, type=T8 {"Module ID"=-1, "abort (F)"=FALSE} ("TCP-Close Connection Argument"), Variant=w362) -> (data=w360:T8, error out=w359:errorcluster)
            n153 = Unbundle By Name(w360) -> ()  [unwired: 2 out]
            n154 = Unbundle By Name(w356) -> ("TCP-ID"=w357:refnum<k5>)
            n155 = TCP Close Connection(connection ID=w357, error in (no error)=w359) -> (error out=w358:errorcluster)  [unwired: 1 in, 1 out]
          }
          frame "---Copy This Frame---" {
            # "Duplicate this frame when creating new messages.  Change this comment in the duplicated frame to describe this message."
            n156 = Merge Errors(w366) -> (w365:errorcluster)
          }
          frame "Verify Retry Time" {
            # "Duplicate this frame when creating new messages.  Change this comment in the duplicated frame to describe this message."
            n157 = Unbundle By Name(w377) -> ("OC Err Time"=w376:timestamp)
            n158 = Get Date/Time In Seconds() -> (seconds since 1Jan1904=w375:timestamp)
            n159 = To Double Precision Float(number=w375) -> (double precision float=w374:dbl)
            n160 = To Double Precision Float(number=w376) -> (double precision float=w373:dbl)
            n161 = Subtract(x=w374, y=w373) -> (x-y=w372:dbl)
            n162 = Greater Or Equal?(x=w372, y=5.0) -> (x >= y?=w367:bool)
            "x >= y?" <- w367
            n163 = case shown="True" w367 {
              tunnel: w370 -> [_ _]
              tunnel: w369 -> [w381 w384]
              tunnel: [w380 w383] -> w368
              frame False {
                n164 = Wait (ms)(milliseconds to wait=u32 100) -> ()  [unwired: 1 out]
                n165 = call-poly <vilib>:"Delacor_lib_QMH_Enqueue Message (poly).vi"("Message"="Verify Retry Time", "Message Queue in"=w381) -> ("error out"=w380:errorcluster)  [unwired: 8 in, 1 out]
              }
              frame True {
                n166 = call-poly <vilib>:"Delacor_lib_QMH_Enqueue Message (poly).vi"("Message"="Retry Open Connection", "Message Queue in"=w384) -> ("error out"=w383:errorcluster)  [unwired: 8 in, 1 out]
              }
            }
            n167 = Merge Errors(w368) -> (w378:errorcluster)
          }
          frame "---Exit and Error Handling---" {
            # "Separator - the following cases handle errors and exit messages."
          }
          frame "Error" {
            # "#CodeRecommended - If the module is running in standalone mode (External Launch = FALSE), this code will pop up an error dialog and call the 'Exit' message if an error occurs. Add more fine-grained error management here."
            # "Error - Check the error message data and respond accordingly. This message is sent by the \"Error Handler\" VIs at the end of each loop in this application."
            n168 = Variant To Data(error in=w399, type=errorcluster {"status"=FALSE, "code"=0, "source"=""} ("error constant"), Variant=w393) -> (data=w388:errorcluster, error out=w397:errorcluster)
            n169 = property on="Property Node" class="Mod Admin"(reference=w392) -> ("Accessors:External Launch"=w391:bool, "Accessors:Module ID"=w389:i32)  [unwired: 1 in, 2 out]
            n170 = local write "error out"(w388) -> ()
            n171 = call "Error Reported.vi"("Error"=w388, "Module ID"=w389) -> ()  [unwired: 9 in, 1 out]
            n172 = case shown="False" w391 {
              tunnel: [w404 _] -> w396
              tunnel: w390 -> [w402 _]
              tunnel: w388 -> [w403 _]
              frame False {
                n173 = disable-structure shown="Default" {
                  disable-tunnel: w403 -> [w405 _]
                  frame condition #0 (active) {
                    # "If the module is running standalone, then pop up an error dialog and call the \"Exit\" message."
                    n174 = call <vilib>:"Simple Error Handler.vi"("error in (no error)"=w405) -> ()  [unwired: 4 in, 5 out]
                  }
                  frame condition #1 {
                    # "To prevent the Simple Error Handler VI from being loaded (e.g. when deploying to a Real-Time target), add the Conditional Disable Symbol \"DQMH_Disable_SEH\" to your project and set it to TRUE."
                  }
                }
                n175 = call-poly <vilib>:"Delacor_lib_QMH_Enqueue Message (poly).vi"("Priority Message? (F)"=TRUE, "Message"="Exit", "Message Queue in"=w402) -> ("error out"=w404:errorcluster)  [unwired: 7 in, 1 out]
              }
              frame True {
                # "If the module was launched externally, calling the Error Reported broadcast VI is the only action performed by the \"Error\" message. The module's caller can then process the error appropriately."
              }
            }
            n176 = Merge Errors(w397, w396) -> (w395:errorcluster)
          }
          frame "Simulate MHL Error" {
            # "#DQMH_HowTo The 'Simulate MHL Error' button  illustrates how the MHL handles errors. This event is instructional in nature and can be removed."
            # "Simulate an error occurring at the MHL"
            n177 = property on="Property Node" class="Mod Admin"(reference=w411) -> ("Accessors:Module ID"=w412:i32)  [unwired: 1 in, 2 out]
            n178 = call "Module Name--constant.vi"("Module ID"=w412) -> ("Module Name"=w407:string)  [unwired: 10 in]
            n179 = Format Into String(format string="Simulated error originating at Message Handling Loop in %s", w407) -> (resulting string=w408:string)  [unwired: 2 in, 1 out]
            n180 = call <vilib>:"Error Cluster From Error Code.vi"("show call chain? (False)"=TRUE, "error message (\"\")"=w408, "error code (0)"=5001) -> ("error out"=w414:errorcluster)  [unwired: 6 in]
            n181 = Merge Errors(w416, w414) -> (w415:errorcluster)
          }
          frame "Exit" {
            w428 = 91  # 91: not all Exit messages will have an argument
            w429 = TRUE  # Stop the VI
            # "Release the message queue reference"
            # "Exit - Exit the application."
            n182 = Variant To Data(error in=w436, type=T5 {"Module ID"=-1, "Origin"="", "Exit via Stop Module Req?"=FALSE, "Wait for Module to stop?"=FALSE} ("Stop Argument"), Variant=w427) -> (data=w424:T5, error out=w432:errorcluster)
            n183 = call <vilib>:"Clear Errors.vi"("error in (no error)"=w432, "specific error code to clear (0: all)"=w428) -> ("error out"=w435:errorcluster)  [unwired: 4 in, 1 out]
            n184 = call-dynamic "Delacor_lib_QMH_Release Message Queue.vi"("error in"=w435, "Message Queue"=w430) -> ("error out"=w434:errorcluster)  [unwired: 9 in]
            n185 = Unbundle By Name(w420) -> ("TCP-ID"=w419:refnum<k5>)
            n186 = TCP Close Connection(connection ID=w419, abort (F)=TRUE) -> (error out=w417:errorcluster)  [unwired: 1 in, 1 out]
            n187 = call <vilib>:"Clear Errors.vi"("error in (no error)"=w417) -> ()  [unwired: 5 in, 2 out]
            n188 = property on="Property Node" class="Mod Admin"(reference=w422) -> ("Accessors:Module ID"=w421:i32)  [unwired: 1 in, 2 out]
            n189 = control-ref of="This VI"() -> (w423:refnum<vi>)
            n190 = call "Handle Exit.vi"("Stop Argument"=w424, "Module Admin in"=w422, "VI reference"=w423) -> ("error out"=w433:errorcluster, "Wait for Stop?"=w425:bool)  [unwired: 7 in]
            n191 = Merge Errors(w434, w433) -> (w431:errorcluster)
            n192 = call "Error Reported.vi"("Error"=w431, "Module ID"=w421) -> ()  [unwired: 9 in, 1 out]
          }
          frame Default {
            # "'Default' case only runs if there is a message that isn't defined in any of the other cases.  Output a programming error."
            n193 = property on="Property Node" class="Mod Admin"(reference=w444) -> ("Accessors:Module ID"=w443:i32)  [unwired: 1 in, 2 out]
            n194 = call "Module Name--constant.vi"("Module ID"=w443) -> ("Module Name"=w437:string)  [unwired: 10 in]
            n195 = Format Into String(format string="The invalid message string \"%s\" was received in the Message Handling Loop for module \"%s\".", w438, w437) -> (resulting string=w440:string)  [unwired: 2 in, 1 out]
            n196 = call <vilib>:"Error Cluster From Error Code.vi"("show call chain? (False)"=TRUE, "error message (\"\")"=w440, "error code (0)"=1) -> ("error out"=w446:errorcluster)  [unwired: 6 in]
            n197 = Merge Errors(w447, w446) -> (w448:errorcluster)
          }
        }
        n198 = call-dynamic "Delacor_lib_QMH_Error Handler - Message Handling Loop.vi"("error in"=w188, "Message Queue in"=w179) -> ("dup error in"=w185:errorcluster)  [unwired: 8 in, 1 out]
      }
    }
    frame Error {
      n199 = call "Synchronize Caller Events.vi"("Module Admin"=w452) -> ("Module Admin out"=w451:refnum<class "Delacor_lib_QMH_Cloneable Module Admin.lvclass">)  [unwired: 9 in, 1 out]
      n200 = property on="Property Node" class="Mod Admin"(reference=w451) -> ("Accessors:Module ID"=w450:i32)  [unwired: 1 in, 2 out]
      n201 = call-dynamic "Delacor_lib_QMH_Release Message Queue.vi"("error in"=w458, "Message Queue"=w449) -> ("error out"=w457:errorcluster)  [unwired: 9 in]
      n202 = call "Module Name--constant.vi"("Module ID"=w450) -> ("Module Name"=w455:string)  [unwired: 10 in]
      n203 = Format Into String(format string="An error occurred during initialization. %s is no longer running.", w455) -> (resulting string=w453:string)  [unwired: 2 in, 1 out]
      n204 = call "Error Reported.vi"("Additional Information"=w453, "Error"=w457, "Module ID"=w450) -> ()  [unwired: 8 in, 1 out]
    }
  }
  n205 = Merge Errors(w17, w16) -> (w18:errorcluster)
  n206 = call "Close Module.vi"("error in"=w18, "Wait for stop?"=w2, "Module Admin in"=w4) -> ("error out"=w14:errorcluster, "External Launch"=w1:bool, "Module Admin out"=w3:refnum<class "Delacor_lib_QMH_Cloneable Module Admin.lvclass">)  [unwired: 6 in]
  n207 = Unregister For Events(event registration refnum=w9, error in=w14) -> (error out=w13:errorcluster)
  "error out" <- w13
  n208 = case "External Launch?" shown="True" w1 {
    tunnel: w13 -> [_ w459]
    frame False {
    }
    frame True {
      n209 = case shown="No Error" w459 {
        frame No Error {
          n210 = invoke class="VI" method="FP.Close"() -> ()  [unwired: 3 in, 3 out]
        }
        frame Error {
          n211 = invoke class="VI" method="FP.Open"("Activate"=TRUE ("Activate?")) -> ()  [unwired: 4 in, 5 out]
        }
      }
    }
  }
  n212 = local write "Module Admin"(w3) -> ()
